vi "AlliGator Is SS2 Dataset HDF5 File.vi"(7 "File Path":path, 9 "Error In":errorcluster) -> (8 "Is SS2 Dataset?":bool, 10 "Error Out":errorcluster)   [LabVIEW 2021, in "AlliGator HDF5.lvlib"]
doc: "Checks wether a HDF5 file is a SS2 dataset file (early version)."
uses:
  AlliGator HDF5.lvlib
  <vilib>/addons/h5labview2/base/lib_path.vi
  <vilib>/addons/h5labview2/base/H5Equery.vi
  <vilib>/addons/h5labview2/base/hid_t.ctl
  <vilib>/addons/h5labview2/dataset/H5Dread.llb/H5Dread.xnode
  <vilib>/addons/h5labview2/file/H5F.lvlib
panel:
  # "see the AlliGator License on the block diagram (Ctrl+E or Window:Show Block Diagram)"
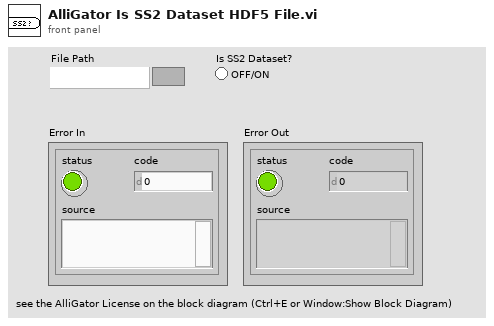
[diagram p1: front panel]
types:
  T1 = typedef "hid_t.ctl" = i64
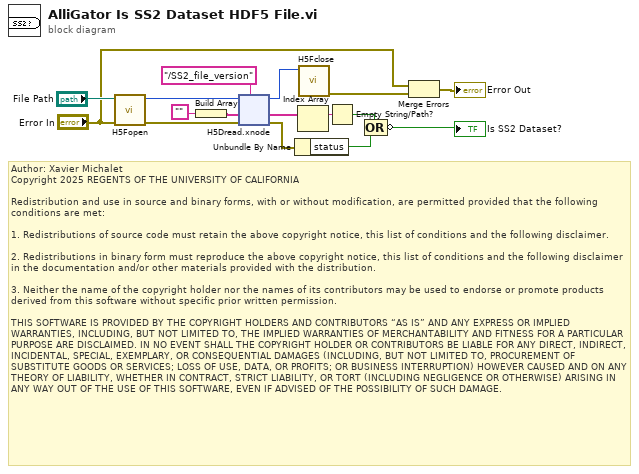
[diagram p0: block diagram]
diagram:
  # "Author: Xavier Michalet\nCopyright 2025 REGENTS OF THE UNIVERSITY OF CALIFORNIA\n\nRedistribution and use in source and binary forms, with or without modification, are permitted provided that the following conditions are met:\n\n1. Redistributions of source code must retain the above copyright notice, this list of conditions and the following disclaimer.\n\n2. Redistributions in binary form must reproduce the above copyright notice, this list of conditions and the following disclaimer in the documentation and/or other materials provided with the distribution.\n\n3. Neither the name of the copyright holder nor the names of its contributors may be used to endorse or promote products derived from this software without specific prior written permission.\n\nTHIS SOFTWARE IS PROVIDED BY THE COPYRIGHT HOLDERS AND CONTRIBUTORS “AS IS” AND ANY EXPRESS OR IMPLIED WARRANTIES, INCLUDING, BUT NOT LIMITED TO, THE IMPLIED WARRANTIES OF MERCHANTABILITY AND FITNESS FOR A PARTICULAR PURPOSE ARE DISCLAIMED. IN NO EVENT SHALL THE COPYRIGHT HOLDER OR CONTRIBUTORS BE LIABLE FOR ANY DIRECT, INDIRECT, INCIDENTAL, SPECIAL, EXEMPLARY, OR CONSEQUENTIAL DAMAGES (INCLUDING, BUT NOT LIMITED TO, PROCUREMENT OF SUBSTITUTE GOODS OR SERVICES; LOSS OF USE, DATA, OR PROFITS; OR BUSINESS INTERRUPTION) HOWEVER CAUSED AND ON ANY THEORY OF LIABILITY, WHETHER IN CONTRACT, STRICT LIABILITY, OR TORT (INCLUDING NEGLIGENCE OR OTHERWISE) ARISING IN ANY WAY OUT OF THE USE OF THIS SOFTWARE, EVEN IF ADVISED OF THE POSSIBILITY OF SUCH DAMAGE."
  n1 = call <vilib>:"H5Fopen.vi"("error in (no error)"="Error In", "path"="File Path") -> ("error out"=w12:errorcluster, "ref out"=w13:T1)  [unwired: 8 in]
  n2 = Build Array("") -> (w14:string[])
  n3 = xnode "H5Dread.xnode"("dataset name (this)"="/SS2_file_version", "error in (no error)"=w12, "default"=w14, "ref in"=w13) -> ("error out"=w9:errorcluster, "data"=w10:string[], "ref out"=w4:T1)  [unwired: 2 in, 1 out]
  n4 = Unbundle By Name(w9) -> ("status"=w7:bool)
  n5 = Index Array(array=w10) -> (element=w5:string)  [unwired: 1 in]
  n6 = call <vilib>:"H5Fclose.vi"("ref"=w4) -> ("error out"=w3:errorcluster)  [unwired: 10 in]
  n7 = Empty String/Path?(string/path=w5) -> (empty?=w8:bool)
  n8 = Compound Arithmetic op=OR(w8, w7) -> (invert →"Is SS2 Dataset?":bool)
  n9 = Merge Errors("Error In", w3) -> (→"Error Out":errorcluster)
